vi "initClass.vi"(8 "error un":errorcluster, 9 "Queue In":T2, 10 "TypeFirmware":T1, 11 "GiaoTiepUART in":refnum<class "GiaoTiepUART.lvclass">) -> (0 "error out":errorcluster, 3 "GiaoTiepUART out":refnum<class "GiaoTiepUART.lvclass">)   [LabVIEW 2014, in "LibraryGcode.lvlib" / "GiaoTiepUART.lvclass"]
uses:
  GiaoTiepUART.lvclass
  control/Queue/QueueCMDandPOS.ctl
  control/Queue/TypeDataPOS.ctl
  control/stateCmdUpdatePara.ctl
  control/TypeFirmwareControl.ctl
  StateMachine_UART.ctl
  control/stateBoardFirmware.ctl
  LibraryGcode.lvlib
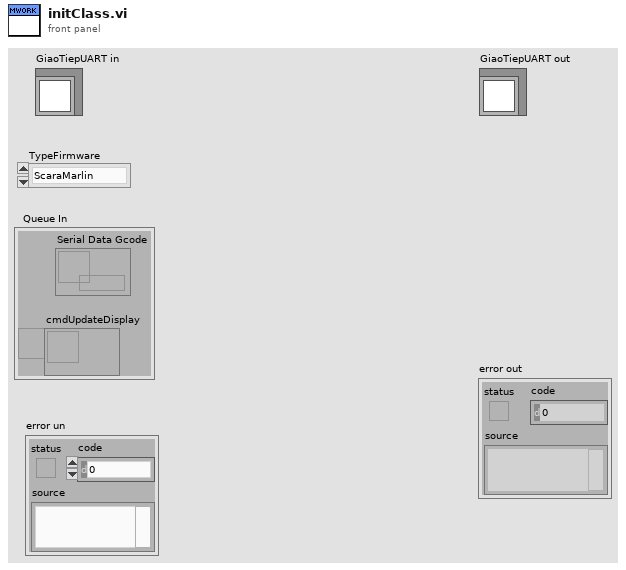
[diagram p1: front panel]
types:
  T1 = typedef "LibraryGcode.lvlib/TypeFirmwareControl.ctl" = enum16{"ScaraMarlin", "CncMarlin", "Mk4Due"}
  T2 = typedef "LibraryGcode.lvlib/QueueCMDandPOS.ctl" = cluster{"Serial Data Gcode":refnum<queue>, "cmdUpdateDisplay":refnum<queue>}
  T3 = typedef "LibraryGcode.lvlib/stateBoardFirmware.ctl" = enum16{"Running", "Waiting", "Pos", "IDLE"}
  T4 = typedef "LibraryGcode.lvlib/GiaoTiepUART.lvclass/StateMachine_UART.ctl" = enum16{"INIT", "WRITE", "READ", "CHECKDATA", "IDLE", "STOP"}
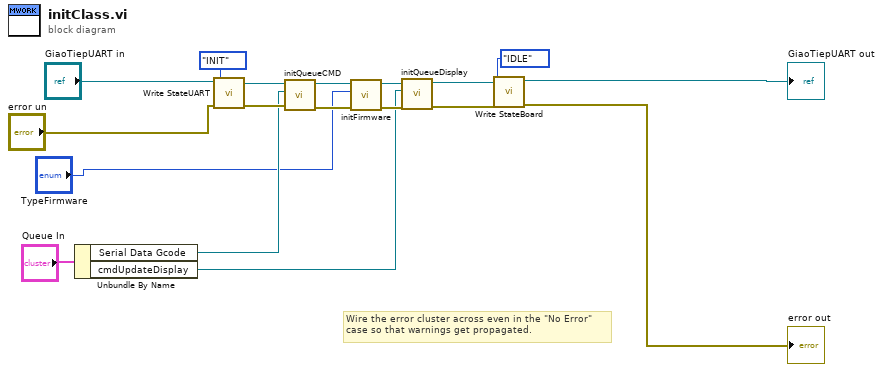
[diagram p0: block diagram]
diagram:
  # "Wire the error cluster across even in the \"No Error\"\ncase so that warnings get propagated."
  n1 = Unbundle By Name("Queue In") -> ("Serial Data Gcode"=w4:refnum<queue>, "cmdUpdateDisplay"=w5:refnum<queue>)
  n2 = call-dynamic "Write StateUART.vi"("error in (no error)"="error un", "STATEUART"=StateMachine_UART."INIT", "GiaoTiepUART in"="GiaoTiepUART in") -> ("error out"=w10:errorcluster, "GiaoTiepUART out"=w14:refnum<class "GiaoTiepUART.lvclass">)  [unwired: 7 in]
  n3 = call-dynamic "initQueueCMD.vi"("error in (no error)"=w10, "Message"=w4, "GiaoTiepUART in"=w14) -> ("error out"=w9:errorcluster, "GiaoTiepUART out"=w13:refnum<class "GiaoTiepUART.lvclass">)  [unwired: 7 in]
  n4 = call-dynamic "initFirmware.vi"("error in (no error)"=w9, "TypeFirmware"="TypeFirmware", "XuLyStringUART in"=w13) -> ("error out"=w8:errorcluster, "XuLyStringUART out"=w12:refnum<class "GiaoTiepUART.lvclass">)  [unwired: 7 in]
  n5 = call-dynamic "initQueueDisplay.vi"("error in (no error)"=w8, "cmdUpdateDisplay"=w5, "XuLyStringUART in"=w12) -> ("error out"=w7:errorcluster, "XuLyStringUART out"=w11:refnum<class "GiaoTiepUART.lvclass">)  [unwired: 7 in]
  n6 = call-dynamic "Write StateBoard.vi"("error in (no error)"=w7, "StatePos"=stateBoardFirmware."IDLE", "XuLyStringUART in"=w11) -> ("error out"=→"error out":errorcluster, "XuLyStringUART out"=→"GiaoTiepUART out":refnum<class "GiaoTiepUART.lvclass">)  [unwired: 7 in]
